vi "Write Setting.vi"(8 "error in (no error)":errorcluster, 9 "Remote Port":u32, 10 "Address":string, 11 "Sync Box in":refnum<class "Sync Box.lvclass">) -> (0 "error out":errorcluster, 3 "Sync Box out":refnum<class "Sync Box.lvclass">)   [LabVIEW 2018, in "Sync Box.lvclass"]
uses:
  Sync Box.lvclass
  Sync Box.lvclass/Sync Box.ctl
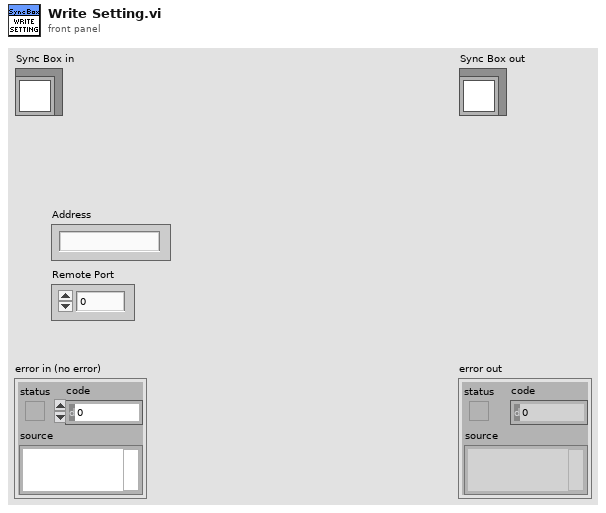
[diagram p1: front panel]
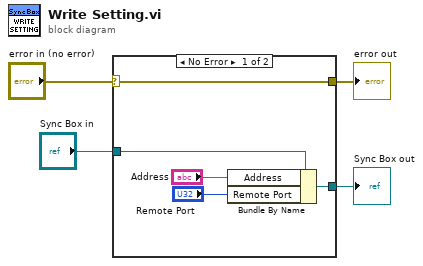
[diagram p0: block diagram]
diagram:
  n1 = case shown="No Error" "error in (no error)" {
    selector: "error in (no error)" -> [w9 w11]
    tunnel: [w9 w11] -> w3
    tunnel: [w7 w10] -> w1
    tunnel: "Sync Box in" -> [w8 w10]
    frame No Error {
      n2 = Bundle By Name(cluster=w8, "Address"="Address", "Remote Port"="Remote Port") -> (w7:refnum<class "Sync Box.lvclass">)
    }
    frame Error {
    }
  }
  "error out" <- w3
  "Sync Box out" <- w1
